vi "Main.vi"(0 "Celsius":dbl, 5 "Stop":bool) -> (4 "Fahrenheit":dbl)   [LabVIEW 2020, in "CelsiusToFarenheit.lvlib"]
doc: "This VI converts Celsius to Fahrenheit."
uses:
  CelsiusToFarenheit.lvlib
panel:
  # "Enter any value to convert from Celsius to Fahrenheit"
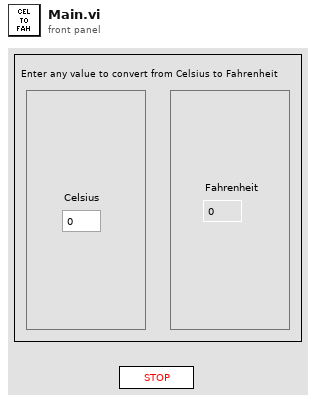
[diagram p1: front panel]
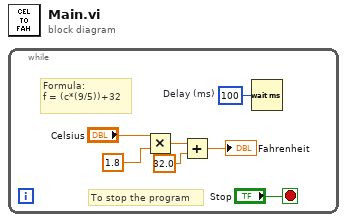
[diagram p0: block diagram]
diagram:
  n1 = while {
    stop <- "Stop" stop-if-true
    w7 = u32 100  # Delay (ms)
    # "To stop the program"
    # "Formula:\nf = (c*(9/5))+32"
    n2 = Multiply(x="Celsius", y=1.8) -> (x*y=w3:dbl)
    n3 = Add(x=w3, y=32.0) -> (x+y=→"Fahrenheit":dbl)
    n4 = Wait (ms)(milliseconds to wait=w7) -> ()  [unwired: 1 out]
  }
